vi "ViewAll.vi"(7 "LabVIEW Web Service Request":refnum<class "Web Request.lvclass">, 10 "ascending":bool=TRUE, 11 "sortMode":u16(ring)=1 items=["Default", "Last Name", "First Name", "Middle Name", "Phone", "Street", "City", "State", "Postal Code", "Favorite"]) -> ()   [LabVIEW 2014]
uses:
  <vilib>/wsapi/Web Request.lvclass
  <vilib>/wsapi/class/subVIs/Set Integer ESP Variable.vi
  <vilib>/wsapi/class/subVIs/Set Boolean ESP Variable.vi
  Libraries/Contact Data/Contact Data.lvlib
panel:
  # "Use the Web Service Request input terminal to call the VIs on the Web Services palette. Do not remove it from the connector pane unless you don't need access to the palette."
  # "Each additional control wired to the connector pane will be available as an input in the URL. To include an indicator in terminal-mode output (the default setting), it must also be wired to the connector pane."
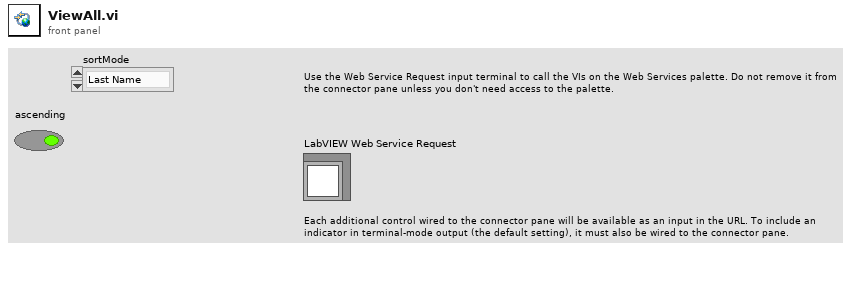
[diagram p1: front panel]
types:
  T1 = typedef "Contact Data.lvlib/Contact.ctl" = cluster{"ID":u32, "UUID":string, "Name":string, "Iteration":i32, "Posit Array":T2[], "Controls":T3, "DestArray":T4[], "SetSpeed":dbl, "Speed":dbl}
  T2 = typedef "Contact Data.lvlib/Position.ctl" = cluster{"X":dbl, "Y":dbl, "Z":dbl}
  T3 = typedef "Contact Data.lvlib/Controls.ctl" = cluster{"throttle":dbl, "brake":dbl, "horn":dbl, "wait":dbl}
  T4 = typedef "Contact Data.lvlib/DestinationCluster.ctl" = cluster{"Desination":string, "DestControls":T5, "Timer":u32, "Set Timer":u32, "Time Stamp":timestamp, "Repeat?":bool, "Optional Data":string, "Distance":dbl}
  T5 = typedef "Contact Data.lvlib/DesinationControls.ctl" = enum16{"Tracker", "Manual", "Stop", "Station DateTime", "Station Timer", "Maintain"}
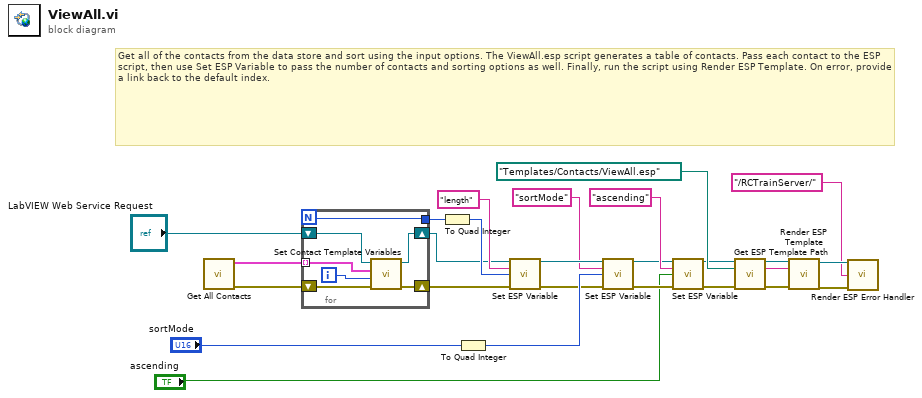
[diagram p0: block diagram]
diagram:
  # "Get all of the contacts from the data store and sort using the input options. The ViewAll.esp script generates a table of contacts. Pass each contact to the ESP script, then use Set ESP Variable to pass the number of contacts and sorting options as well. Finally, run the script using Render ESP Template. On error, provide a link back to the default index."
  n1 = call "Get All Contacts.vi"() -> ("error out"=w20:errorcluster, "Contacts"=w19:T1[])  [unwired: 10 in]
  n2 = for {
    N -> [w27]
    tunnel: w19 -> [w32] mode=indexing
    shift-right: [w29] -> w26
    shift-left: w20 -> [w30]
    shift-right: [w28] -> w22
    shift-left: "LabVIEW Web Service Request" -> [w33]
    tunnel: [w27] -> w24
    i -> [w31]
    n3 = call "Set Contact Template Variables.vi"("error in (no error)"=w30, "Index (none)"=w31, "Contact"=w32, "LabVIEW Web Service Request"=w33) -> ("error out"=w29:errorcluster, "LabVIEW Web Service Request out"=w28:refnum<class "Web Request.lvclass">)  [unwired: 6 in]
  }
  n4 = To Quad Integer(1:w24) -> (0:w23:i64)
  n5 = To Quad Integer(1:"sortMode") -> (0:w8:i64)
  n6 = call-poly <vilib>:"Set ESP Variable.vi"("LabVIEW Web Service Request"=w22, "key"="length", "value"=w23, "error in (no error)"=w26) -> ("LabVIEW Web Service Request out"=w5:refnum<class "Web Request.lvclass">, "error out"=w4:errorcluster)  [unwired: 10 in]
  n7 = call-poly <vilib>:"Set ESP Variable.vi"("LabVIEW Web Service Request"=w5, "key"="sortMode", "value"=w8, "error in (no error)"=w4) -> ("LabVIEW Web Service Request out"=w7:refnum<class "Web Request.lvclass">, "error out"=w11:errorcluster)  [unwired: 10 in]
  n8 = call-poly <vilib>:"Set ESP Variable.vi"("LabVIEW Web Service Request"=w7, "key"="ascending", "value"="ascending", "error in (no error)"=w11) -> ("LabVIEW Web Service Request out"=w2:refnum<class "Web Request.lvclass">, "error out"=w3:errorcluster)  [unwired: 10 in]
  n9 = call "Get ESP Template Path.vi"("LabVIEW Web Service Request"=w2, "Relative Template Path"=path "Templates/Contacts/ViewAll.esp", "error in (no error)"=w3) -> ("LabVIEW Web Service Request out"=w18:refnum<class "Web Request.lvclass">, "Template Name"=w15:string, "error out"=w17:errorcluster)  [unwired: 10 in]
  n10 = call <vilib>:"Render ESP Template.vi"("LabVIEW Web Service Request"=w18, "espName"=w15, "error in (no error)"=w17) -> ("LabVIEW Web Service Request out"=w13:refnum<class "Web Request.lvclass">, "error out"=w14:errorcluster)  [unwired: 11 in]
  n11 = call "Render ESP Error Handler.vi"("LabVIEW Web Service Request"=w13, "Link"="/RCTrainServer/", "error in (no error)"=w14) -> ()  [unwired: 11 in, 2 out]
